vi "db_advanced_nonVoid.vi"(0 "UDL FILEPATH":path, 2 "QUERIES":string[](array[string]), 5 "ERROR IN":errorcluster) -> (14 "LIST OF RECORDSET":string[][][](array[string]), 16 "SUCCESS?":bool, 17 "LAST QUERY":i32)   [LabVIEW 2018, in "db_lib R3.lvlib"]
uses:
  db_lib R3.lvlib
  <vilib>/addons/database/Connection.llb/DB Tools Open Connec (Path).vi
  <vilib>/addons/database/Connection.llb/Conn Execute.vi
  <vilib>/addons/database/Recordset.llb/Rec Fetch Recordset Data (R).vi
  <vilib>/addons/database/Recordset.llb/Rec Destroy - Connection.vi
  <vilib>/addons/database/_DB Variant To Data/Database Variant To Data.xnode
  <vilib>/addons/database/NI_Database_API.lvlib
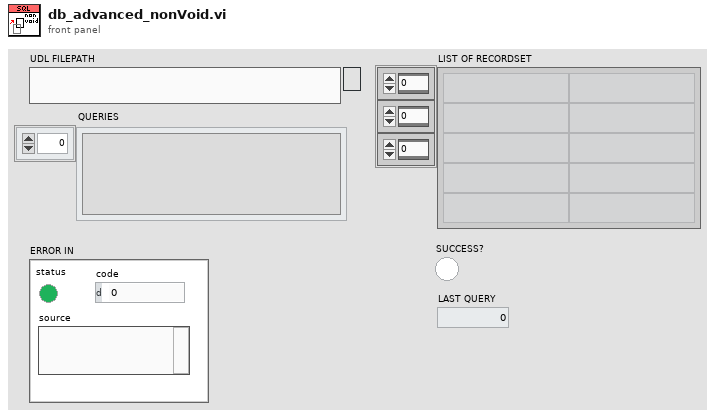
[diagram p1: front panel]
types:
  T1 = typedef "NI_Database_API.lvlib/Conn ObjectReference.ctl" = refnum<k1>
  T2 = typedef "NI_Database_API.lvlib/Rec ObjectReference.ctl" = refnum<k1>
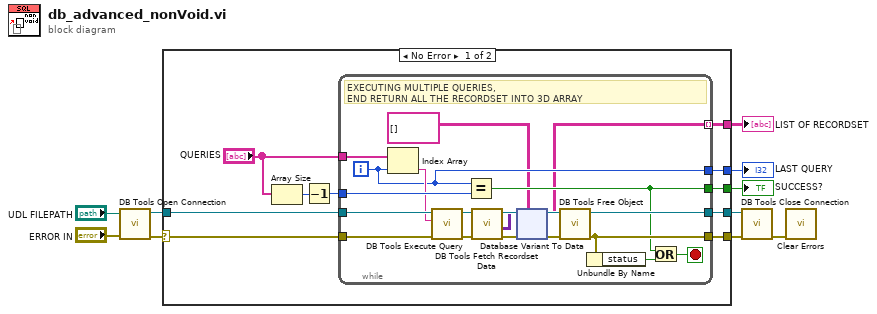
[diagram p0: block diagram]
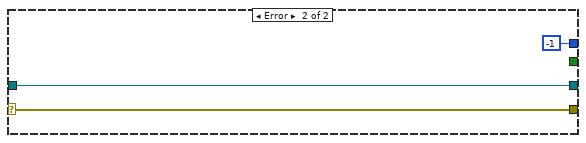
[diagram p2: hidden frame]
diagram:
  n1 = call-poly <vilib>:"DB Tools Open Connection.vi"("error in (no error)"="ERROR IN", "connection information"="UDL FILEPATH") -> ("error out"=w4:errorcluster, "connection reference"=w10:T1)  [unwired: 6 in]
  n2 = case shown="No Error" w4 {
    selector: w4 -> [w17 w84]
    tunnel: w10 -> [w20 w85]
    tunnel: [w19 w85] -> w9
    tunnel: [w18 w84] -> w8
    tunnel: [w13 _] -> w3
    tunnel: [w12 -1] -> w2
    tunnel: [w11 _] -> w1
    frame No Error {
      n3 = Array Size(array="QUERIES") -> (size(s)=w15:i32)
      n4 = Decrement(x=w15) -> (x-1=w14:i32)
      n5 = while {
        tunnel: w20 -> [w39]
        tunnel: [w35] -> w19
        tunnel: [w27] -> w18
        tunnel: w17 -> [w32]
        tunnel: "QUERIES" -> [w30]
        tunnel: w14 -> [w29]
        tunnel: [w24] -> w13
        tunnel: [w23] -> w12
        tunnel: [w21] -> w11 mode=indexing
        i -> [w23]
        stop <- w25 stop-if-true
        # "EXECUTING MULTIPLE QUERIES,\nEND RETURN ALL THE RECORDSET INTO 3D ARRAY"
        n6 = Index Array(array=w30, index=w23) -> (element=w28:string)
        n7 = call-poly <vilib>:"DB Tools Execute Query.vi"("error in (no error)"=w32, "SQL query"=w28, "connection reference"=w39) -> ("error out"=w37:errorcluster, "recordset reference"=w38:T2)  [unwired: 5 in]
        n8 = Equal?(x=w23, y=w29) -> (x = y?=w24:bool)
        n9 = call-poly <vilib>:"DB Tools Fetch Recordset Data.vi"("error in (no error)"=w37, "recordset reference"=w38) -> ("error out"=w34:errorcluster, "recordset data"=w31:variant[][], "recordset reference out"=w36:T2)  [unwired: 3 in]
        n10 = xnode "Database Variant To Data"("database variant"=w31, "error in (no error)"=w34, "type"=string[][] []) -> ("data"=w21:string[][], "error out"=w33:errorcluster)
        n11 = call-poly <vilib>:"DB Tools Free Object.vi"("error in (no error)"=w33, "recordset reference"=w36) -> ("error out"=w27:errorcluster, "connection reference"=w35:T1)  [unwired: 8 in]
        n12 = Unbundle By Name(w27) -> ("status"=w26:bool)
        n13 = Or(x=w24, y=w26) -> (x .or. y?=w25:bool)
      }
    }
    frame Error {
    }
  }
  "LIST OF RECORDSET" <- w1
  "SUCCESS?" <- w3
  "LAST QUERY" <- w2
  n14 = call <vilib>:"DB Tools Close Connection.vi"("error in (no error)"=w8, "connection reference"=w9) -> ("error out"=w5:errorcluster)  [unwired: 5 in]
  n15 = call <vilib>:"Clear Errors.vi"("error in (no error)"=w5) -> ()  [unwired: 5 in, 2 out]
